vi "Send Raw Pixel to FPGA.vi"(7 "file path (use dialog)":path=path "\\\\vmware-host\\Shared Folders/Downloads/pug.bin", 8 "error in":errorcluster, 11 "FPGA VI Reference Out":T1) -> (0 "error out":errorcluster, 3 "FPGA VI Reference Out 2":T1)   [LabVIEW 2019]
uses:
  TypeDefs/FPGA Reference.ctl
  <vilib>/Utility/error.llb/Error Cluster From Error Code.vi
  <vilib>/rvi/errors/niLvFpgaAdjustHostInterfaceError.vi
  <vilib>/rvi/interface/nirviMethod/nirviMethod.xnode
  FPGA Bitfiles/adafruitlcdsom_FPGATarget_FPGAMain_K7l+4zj6vFY.lvbitx
  FPGA Main.vi
  <vilib>/FPGAPlugInAG/sbRIO-9651/niLvFpga_WriteFifo_sbRIO-9651.vi
  <vilib>/rvi/errors/niLvFpgaMergeErrorWithErrorCode.vi
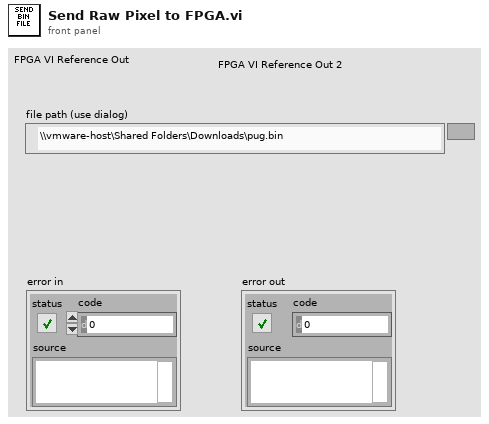
[diagram p1: front panel]
types:
  T1 = typedef "FPGA Reference.ctl" = refnum<k20>
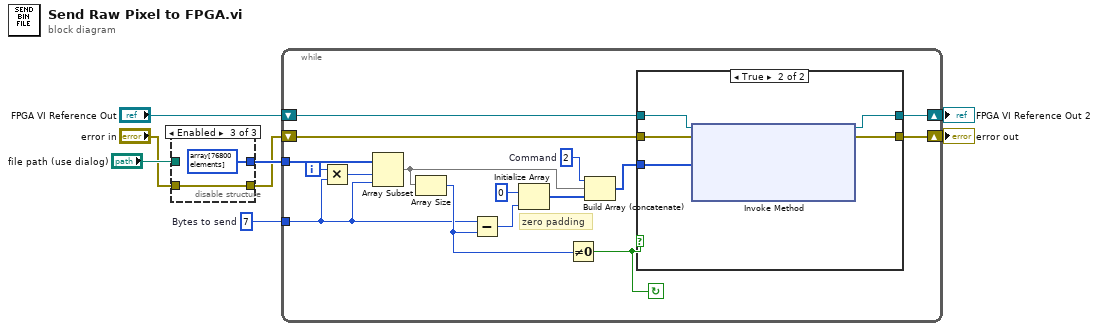
[diagram p0: block diagram]
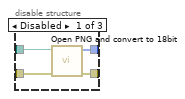
[diagram p2: hidden frame]
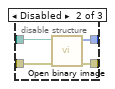
[diagram p3: hidden frame]
diagram:
  w3 = 7  # Bytes to send
  n1 = disable-structure shown="Enabled" {
    disable-tunnel: "file path (use dialog)" -> [w12 w16 _]
    disable-tunnel: [w11 w15 u16[] array[76800 elements] ("data")] -> w4
    disable-tunnel: "error in" -> [w10 w14 w17]
    disable-tunnel: [w9 w13 w17] -> w1
    frame Disabled {
      n2 = call "Open PNG and convert to 18bit.vi"("error in"=w10, "file path (use dialog)"=w12) -> ("error out"=w9:errorcluster, "data"=w11:u16[])  [unwired: 8 in]
    }
    frame Disabled {
      n3 = call "Open binary image.vi"("error in"=w14, "file path (use dialog)"=w16) -> ("error out"=w13:errorcluster, "data"=w15:u16[])  [unwired: 8 in]
    }
    frame Enabled {
    }
  }
  n4 = while {
    shift-right: [w33] -> w7
    shift-left: "FPGA VI Reference Out" -> [w34]
    shift-right: [w32] -> w6
    shift-left: w1 -> [w31]
    tunnel: w4 -> [w28]
    tunnel: w3 -> [w19]
    i -> [w27]
    stop <- w22 continue-if-true
    w30 = u16 2  # Command
    # "zero padding"
    n5 = Multiply(x=w27, y=w19) -> (x*y=w26:i32)
    n6 = Array Subset(array=w28, index=w26, length=w19) -> (w25:u16[])
    n7 = Array Size(array=w25) -> (size(s)=w21:i32)
    n8 = Subtract(x=w19, y=w21) -> (x-y=w20:i32)
    n9 = Initialize Array(u16 0 ("X"), w20) -> (w23:u16[])
    n10 = Not Equal To 0?(x=w21) -> (x != 0?=w22:bool)
    n11 = Build Array (concatenate)(w30, w25, w23) -> (w29:u16[])
    n12 = case shown="True" w22 {
      tunnel: w34 -> [w36 w41]
      tunnel: [w36 w40] -> w33
      tunnel: [w35 w39] -> w32
      tunnel: w31 -> [w35 w38]
      tunnel: w29 -> [_ w37]
      frame False {
      }
      frame True {
        n13 = xnode "Invoke Method"("FPGA VI Reference In"=w41, "error in"=w38, "Data"=w37) -> ("FPGA VI Reference Out"=w40:T1, "error out"=w39:errorcluster)  [unwired: 1 in, 1 out]
      }
    }
  }
  "FPGA VI Reference Out 2" <- w7
  "error out" <- w6
